vi "FourwayTrafficLights.vi"() -> ()   [LabVIEW 2015]
panel:
  in  "Activate":bool
  in  "Stop":bool
  out "G_D":bool
  out "Y_D":bool
  out "R_D":bool
  out "G_B":bool
  out "Y_B":bool
  out "R_B":bool
  out "G_C":bool
  out "Y_C":bool
  out "R_C":bool
  out "R_A":bool
  out "Y_A":bool
  out "G_A":bool
  # "Four way Traffic Light System"
  # "C"
  # "A"
  # "B"
  # "D"
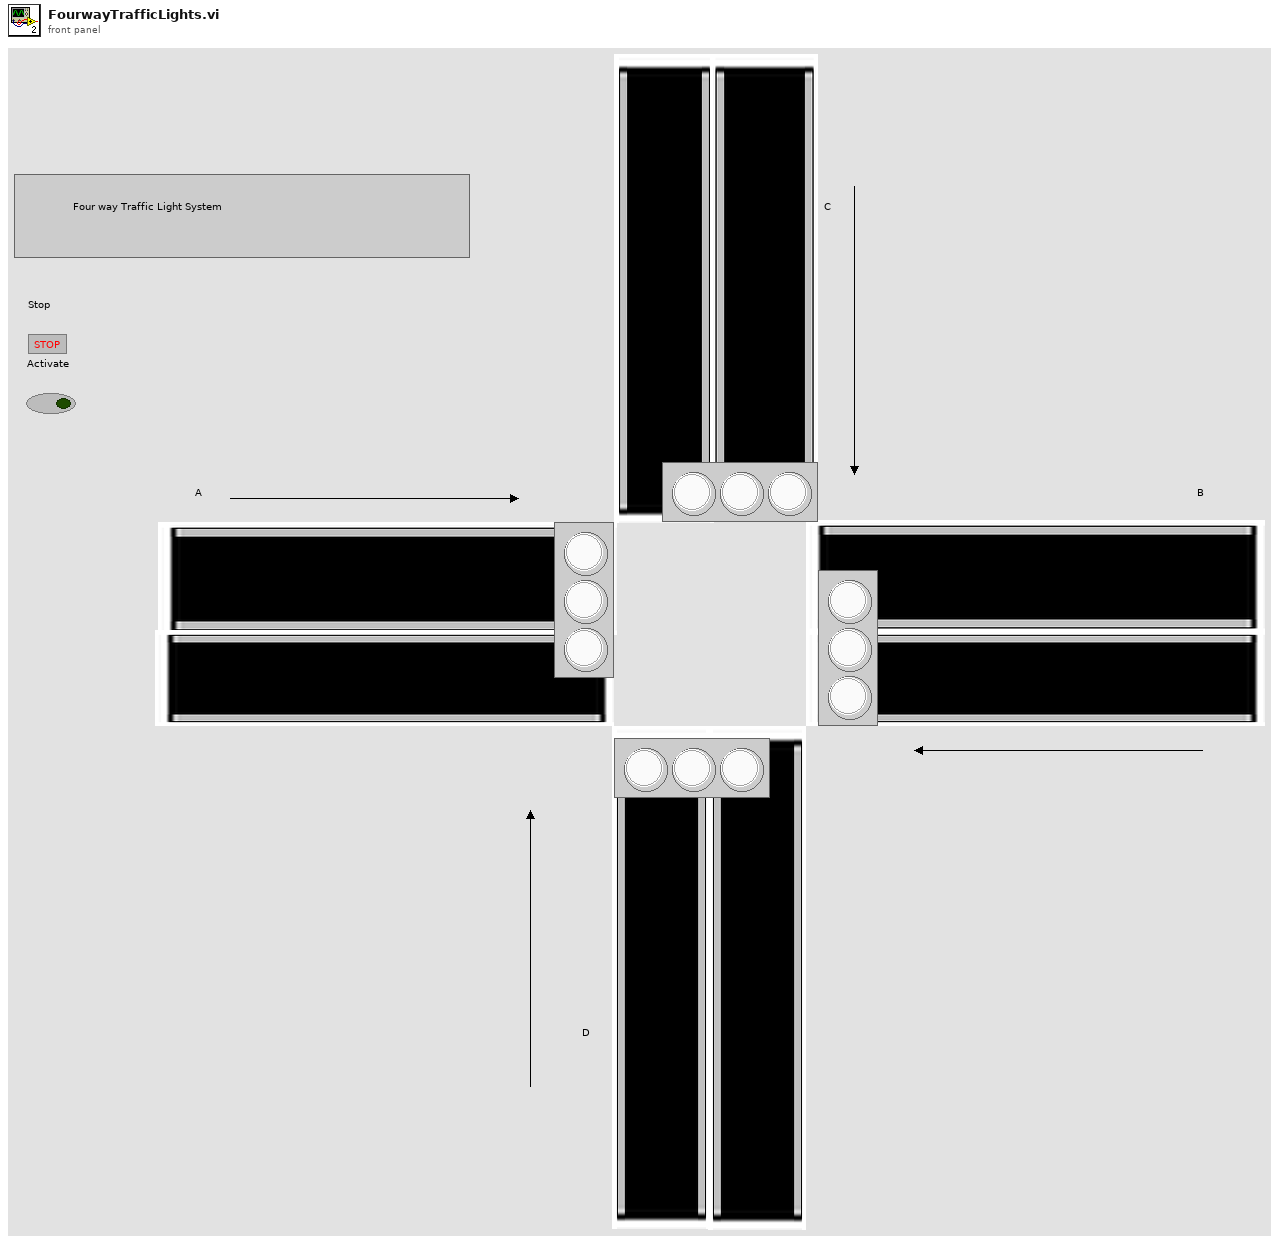
[diagram p1: front panel]
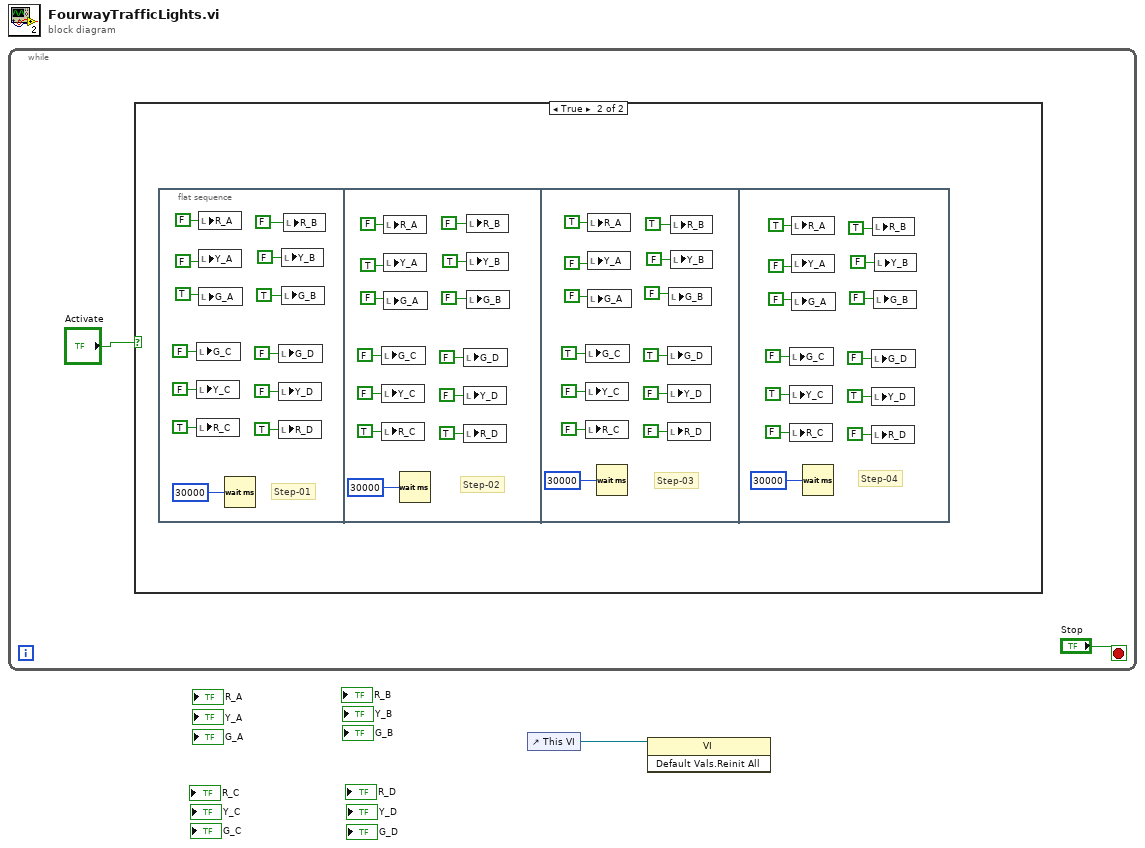
[diagram p0: block diagram]
diagram:
  n1 = while {
    stop <- "Stop" stop-if-true
    n2 = case shown="True" "Activate" {
      frame False {
      }
      frame True {
        n3 = flat-sequence {
          frame #0 {
            # "Step-01"
            n4 = local write "G_C"(FALSE ("G_C")) -> ()
            n5 = local write "Y_C"(FALSE ("Y_C")) -> ()
            n6 = local write "R_C"(TRUE ("R_C")) -> ()
            n7 = local write "R_A"(FALSE ("R_A")) -> ()
            n8 = local write "Y_A"(FALSE ("Y_A")) -> ()
            n9 = local write "G_A"(TRUE ("G_A")) -> ()
            n10 = Wait (ms)(milliseconds to wait=u32 30000 ("millisecond timer value")) -> ()  [unwired: 1 out]
            n11 = local write "G_D"(FALSE ("G_D")) -> ()
            n12 = local write "Y_D"(FALSE ("Y_D")) -> ()
            n13 = local write "R_D"(TRUE ("R_D")) -> ()
            n14 = local write "Y_B"(FALSE ("Y_B")) -> ()
            n15 = local write "G_B"(TRUE ("G_B")) -> ()
            n16 = local write "R_B"(FALSE ("R_B")) -> ()
          }
          frame #1 {
            # "Step-02"
            n17 = local write "G_C"(FALSE ("G_C")) -> ()
            n18 = local write "Y_C"(FALSE ("Y_C")) -> ()
            n19 = local write "R_C"(TRUE ("R_C")) -> ()
            n20 = local write "R_A"(FALSE ("R_A")) -> ()
            n21 = local write "Y_A"(TRUE ("Y_A")) -> ()
            n22 = local write "G_A"(FALSE ("G_A")) -> ()
            n23 = Wait (ms)(milliseconds to wait=u32 30000 ("millisecond timer value")) -> ()  [unwired: 1 out]
            n24 = local write "G_D"(FALSE ("G_D")) -> ()
            n25 = local write "Y_D"(FALSE ("Y_D")) -> ()
            n26 = local write "R_D"(TRUE ("R_D")) -> ()
            n27 = local write "R_B"(FALSE ("R_B")) -> ()
            n28 = local write "Y_B"(TRUE ("Y_B")) -> ()
            n29 = local write "G_B"(FALSE ("G_B")) -> ()
          }
          frame #2 {
            # "Step-03"
            n30 = local write "G_C"(TRUE ("G_C")) -> ()
            n31 = local write "Y_C"(FALSE ("Y_C")) -> ()
            n32 = local write "R_C"(FALSE ("R_C")) -> ()
            n33 = local write "R_A"(TRUE ("R_A")) -> ()
            n34 = local write "Y_A"(FALSE ("Y_A")) -> ()
            n35 = local write "G_A"(FALSE ("G_A")) -> ()
            n36 = Wait (ms)(milliseconds to wait=u32 30000 ("millisecond timer value")) -> ()  [unwired: 1 out]
            n37 = local write "G_D"(TRUE ("G_D")) -> ()
            n38 = local write "Y_D"(FALSE ("Y_D")) -> ()
            n39 = local write "R_D"(FALSE ("R_D")) -> ()
            n40 = local write "G_B"(FALSE ("G_B")) -> ()
            n41 = local write "R_B"(TRUE ("R_B")) -> ()
            n42 = local write "Y_B"(FALSE ("Y_B")) -> ()
          }
          frame #3 {
            # "Step-04"
            n43 = local write "G_C"(FALSE ("G_C")) -> ()
            n44 = local write "Y_C"(TRUE ("Y_C")) -> ()
            n45 = local write "R_C"(FALSE ("R_C")) -> ()
            n46 = local write "R_A"(TRUE ("R_A")) -> ()
            n47 = local write "Y_A"(FALSE ("Y_A")) -> ()
            n48 = local write "G_A"(FALSE ("G_A")) -> ()
            n49 = Wait (ms)(milliseconds to wait=u32 30000 ("millisecond timer value")) -> ()  [unwired: 1 out]
            n50 = local write "G_D"(FALSE ("G_D")) -> ()
            n51 = local write "Y_D"(TRUE ("Y_D")) -> ()
            n52 = local write "R_D"(FALSE ("R_D")) -> ()
            n53 = local write "R_B"(TRUE ("R_B")) -> ()
            n54 = local write "G_B"(FALSE ("G_B")) -> ()
            n55 = local write "Y_B"(FALSE ("Y_B")) -> ()
          }
        }
      }
    }
  }
  n56 = control-ref of="This VI"() -> (w1:refnum<vi>)
  n57 = invoke class="VI" method="Default Vals.Reinit All"(reference=w1) -> ()  [unwired: 2 in, 3 out]
